vi "Scan Setup.vi"(8 "error in (no error)":errorcluster, 11 "Magnetic Field Lakeshore Continuous in":refnum<class "Magnetic Field Lakeshore Continuous.lvclass">) -> (0 "error out":errorcluster, 3 "Magnetic Field Lakeshore Continuous out":refnum<class "Magnetic Field Lakeshore Continuous.lvclass">)   [LabVIEW 2023, in "Magnetic Field Lakeshore Continuous.lvclass"]
doc: "Configure the Instrument based on the class member fields. This step comes after the user has closed the \"Scan Setup\" window and before the actual scan -- so instruments are configured with the user's specified settings."
uses:
  Magnetic Field Lakeshore Continuous.lvclass
  Magnetic Field Lakeshore Continuous.lvclass/Magnetic Field Lakeshore Continuous.ctl
  Scanner/Scanner.lvclass
  Instruments/Utility Classes/Scannable/Scannable.lvclass
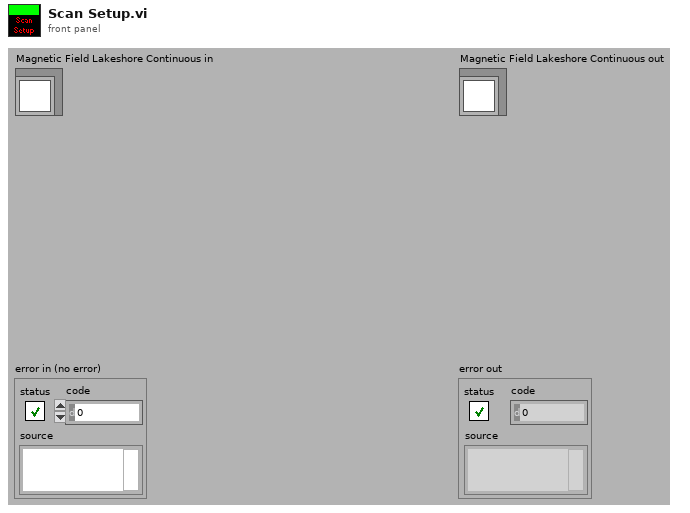
[diagram p1: front panel]
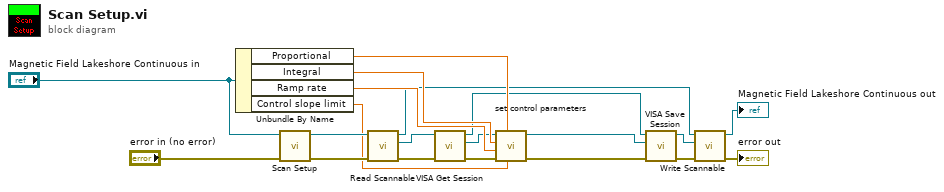
[diagram p0: block diagram]
diagram:
  n1 = Unbundle By Name("Magnetic Field Lakeshore Continuous in") -> ("Proportional"=w9:dbl, "Integral"=w10:dbl[unit], "Ramp rate"=w11:dbl[unit], "Control slope limit"=w12:dbl[unit])
  n2 = call-parent "Scan Setup.vi"("error in (no error)"="error in (no error)", "Scanner in"="Magnetic Field Lakeshore Continuous in") -> ("error out"=w13:errorcluster, "Scanner out"=w19:refnum<class "Magnetic Field Lakeshore Continuous.lvclass">)  [unwired: 8 in]
  n3 = call-dynamic "Read Scannable.vi"("error in (no error)"=w13, "Scanner.lvclass in"=w19) -> ("error out"=w17:errorcluster, "Scannable.lvclass"=w6:refnum<class "Scannable.lvclass">, "Scanner.lvclass out"=w3:refnum<class "Magnetic Field Lakeshore Continuous.lvclass">)  [unwired: 7 out]
  n4 = call-dynamic "VISA Get Session.vi"("error in (no error)"=w17, "Instrument.lvclass in"=w6) -> ("error out"=w2:errorcluster, "VISA Resource Name"=w1:refnum<visa-resource-name>, "Instrument.lvclass out"=w7:refnum<class "Scannable.lvclass">)  [unwired: 7 out]
  n5 = call "set control parameters.vi"("Control slope limit (10 V/min)"=w12, "Proportional (10)"=w9, "error in (no error)"=w2, "Ramp rate (3500 Gs/min)"=w11, "Integral (1 s)"=w10, "VISA session"=w1) -> ("error out"=w16:errorcluster, "dup VISA session"=w8:refnum<visa-resource-name>)  [unwired: 4 in]
  n6 = call-dynamic "VISA Save Session.vi"("error in (no error)"=w16, "VISA Resource Name"=w8, "Instrument.lvclass in"=w7) -> ("error out"=w15:errorcluster, "Instrument.lvclass out"=w5:refnum<class "Scannable.lvclass">)  [unwired: 7 out]
  n7 = call-dynamic "Write Scannable.vi"("error in (no error)"=w15, "Scannable.lvclass"=w5, "Scanner.lvclass in"=w3) -> ("error out"=→"error out":errorcluster, "Scanner.lvclass out"=→"Magnetic Field Lakeshore Continuous out":refnum<class "Magnetic Field Lakeshore Continuous.lvclass">)  [unwired: 7 out]
